vi "VerifyResponse.vi"(8 "error in":errorcluster, 9 "Address #":u8, 10 "Command #":u8, 11 "Data In":T1) -> (0 "error out":errorcluster, 3 "Data out":T1)   [LabVIEW 2020, in "driver_flodx_ph_probe.lvlib"]
uses:
  <instrlib>/RxnRover/FloDx Ph Probe Driver/driver_flodx_ph_probe.lvlib
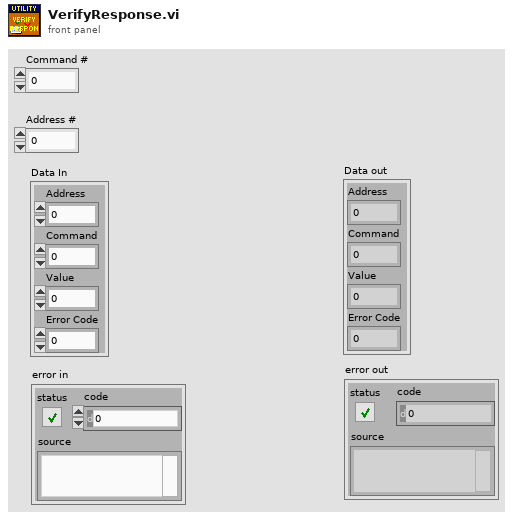
[diagram p1: front panel]
types:
  T1 = cluster{"Address":u32, "Command":u32, "Value":dbl, "Error Code":u32}
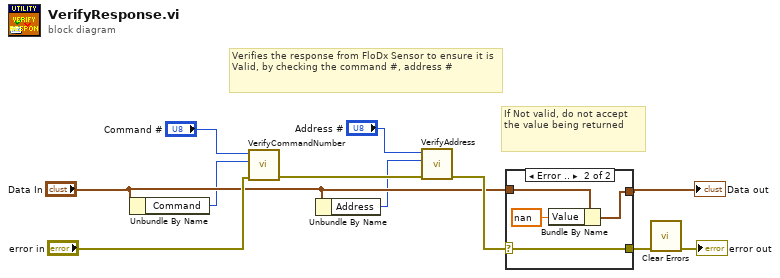
[diagram p0: block diagram]
diagram:
  # "If Not valid, do not accept the value being returned"
  # "Verifies the response from FloDx Sensor to ensure it is Valid, by checking the command #, address #"
  n1 = Unbundle By Name("Data In") -> ("Command"=w4:u32)
  n2 = call <instrlib>:"VerifyCommandNumber.vi"("error in"="error in", "Command #(From Response)"=w4, "Command #"="Command #") -> ("error out"=w10:errorcluster)  [unwired: 8 in]
  n3 = Unbundle By Name("Data In") -> ("Address"=w3:u32)
  n4 = call <instrlib>:"VerifyAddress.vi"("error in"=w10, "Address(From Response)"=w3, "Address #"="Address #") -> ("error out"=w9:errorcluster)  [unwired: 8 in]
  n5 = case shown="Error .." w9 {
    selector: w9 -> [w13 w17]
    tunnel: [w13 w17] -> w2
    tunnel: [w12 w16] -> w7
    tunnel: "Data In" -> [w12 w15]
    frame No Error {
    }
    frame Error {
      n6 = Bundle By Name(cluster=w15, "Value"=nan) -> (w16:T1)
    }
  }
  "Data out" <- w7
  n7 = call <vilib>:"Clear Errors.vi"("error in (no error)"=w2) -> ("error out"=→"error out":errorcluster)  [unwired: 5 in, 1 out]
